vi "getCodeElementsFromApplicationXMLFile.vi"(2 "error in (no error)":errorcluster, 3 "Node":refnum<k20>) -> (0 "error out":errorcluster, 1 "TextElements":T1)   [LabVIEW 2010]
uses:
  Program Files/National Instruments/LabVIEW 2010/resource/objmgr/DOMUserDefRef.rc
panel:
  out "XML":string
  # "从应用层指令中查找出返回数据的类型、指令、控制码等信息"
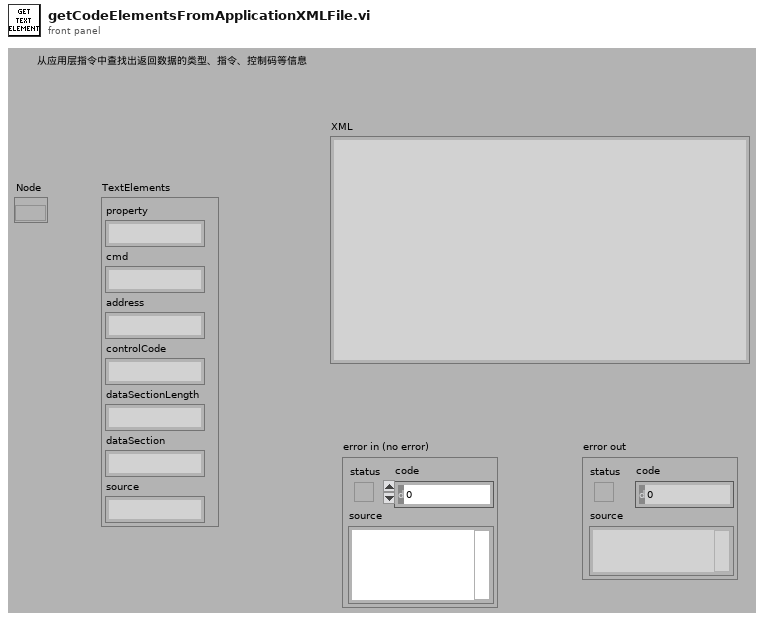
[diagram p1: front panel]
types:
  T1 = cluster{"property":string, "cmd":string, "address":string, "controlCode":string, "dataSectionLength":string, "dataSection":string, "source":string}
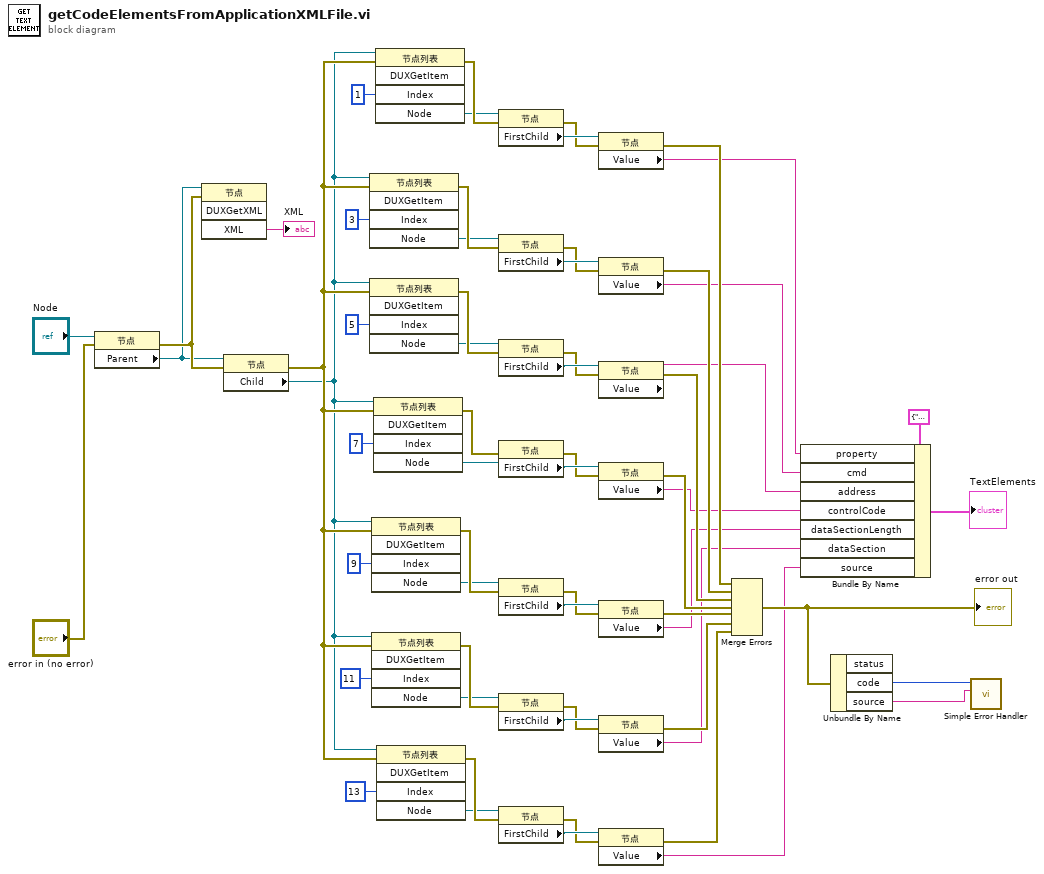
[diagram p0: block diagram]
diagram:
  n1 = property class="节点"(reference="Node", error in="error in (no error)") -> (error out=w55:errorcluster, "Parent"=w15:refnum<k20>)  [unwired: 1 out]
  n2 = invoke class="节点" method="DUXGetXML"(reference=w15, error in=w55) -> ("XML"=→"XML":string)  [unwired: 2 in, 3 out]
  n3 = property class="节点"(reference=w15, error in=w55) -> (error out=w54:errorcluster, "Child"=w22:refnum<k20>)  [unwired: 1 out]
  n4 = invoke class="节点列表" method="DUXGetItem"(reference=w22, error in=w54, "Index"=3) -> (error out=w57:errorcluster, "Node"=w24:refnum<k20>)  [unwired: 2 in, 3 out]
  n5 = invoke class="节点列表" method="DUXGetItem"(reference=w22, error in=w54, "Index"=5) -> (error out=w56:errorcluster, "Node"=w25:refnum<k20>)  [unwired: 2 in, 3 out]
  n6 = invoke class="节点列表" method="DUXGetItem"(reference=w22, error in=w54, "Index"=9) -> (error out=w59:errorcluster, "Node"=w29:refnum<k20>)  [unwired: 2 in, 3 out]
  n7 = invoke class="节点列表" method="DUXGetItem"(reference=w22, error in=w54, "Index"=11) -> (error out=w60:errorcluster, "Node"=w31:refnum<k20>)  [unwired: 2 in, 3 out]
  n8 = invoke class="节点列表" method="DUXGetItem"(reference=w22, error in=w54, "Index"=7) -> (error out=w11:errorcluster, "Node"=w27:refnum<k20>)  [unwired: 2 in, 3 out]
  n9 = invoke class="节点列表" method="DUXGetItem"(reference=w22, error in=w54, "Index"=1) -> (error out=w58:errorcluster, "Node"=w35:refnum<k20>)  [unwired: 2 in, 3 out]
  n10 = invoke class="节点列表" method="DUXGetItem"(reference=w22, error in=w54, "Index"=13) -> (error out=w61:errorcluster, "Node"=w33:refnum<k20>)  [unwired: 2 in, 3 out]
  n11 = property class="节点"(reference=w35, error in=w58) -> (error out=w10:errorcluster, "FirstChild"=w36:refnum<k20>)  [unwired: 1 out]
  n12 = property class="节点"(reference=w24, error in=w57) -> (error out=w9:errorcluster, "FirstChild"=w23:refnum<k20>)  [unwired: 1 out]
  n13 = property class="节点"(reference=w25, error in=w56) -> (error out=w8:errorcluster, "FirstChild"=w26:refnum<k20>)  [unwired: 1 out]
  n14 = property class="节点"(reference=w27, error in=w11) -> (error out=w7:errorcluster, "FirstChild"=w28:refnum<k20>)  [unwired: 1 out]
  n15 = property class="节点"(reference=w29, error in=w59) -> (error out=w6:errorcluster, "FirstChild"=w30:refnum<k20>)  [unwired: 1 out]
  n16 = property class="节点"(reference=w31, error in=w60) -> (error out=w5:errorcluster, "FirstChild"=w32:refnum<k20>)  [unwired: 1 out]
  n17 = property class="节点"(reference=w33, error in=w61) -> (error out=w4:errorcluster, "FirstChild"=w34:refnum<k20>)  [unwired: 1 out]
  n18 = property class="节点"(reference=w36, error in=w10) -> (error out=w46:errorcluster, "Value"=w38:string)  [unwired: 1 out]
  n19 = property class="节点"(reference=w23, error in=w9) -> (error out=w51:errorcluster, "Value"=w39:string)  [unwired: 1 out]
  n20 = property class="节点"(reference=w26, error in=w8) -> (error out=w50:errorcluster, "Value"=w40:string)  [unwired: 1 out]
  n21 = property class="节点"(reference=w28, error in=w7) -> (error out=w49:errorcluster, "Value"=w41:string)  [unwired: 1 out]
  n22 = property class="节点"(reference=w30, error in=w6) -> (error out=w52:errorcluster, "Value"=w42:string)  [unwired: 1 out]
  n23 = property class="节点"(reference=w32, error in=w5) -> (error out=w48:errorcluster, "Value"=w43:string)  [unwired: 1 out]
  n24 = property class="节点"(reference=w34, error in=w4) -> (error out=w47:errorcluster, "Value"=w44:string)  [unwired: 1 out]
  n25 = Merge Errors(w46, w51, w50, w49, w52, w48, w47) -> (w53:errorcluster)
  "error out" <- w53
  n26 = Bundle By Name(cluster=T1 {"property"="读通信地址", "cmd"="主站请求帧", "address"="############", "controlCode"="13", "dataSectionLength"="00", "dataSection"="无", "source"="主站"} ("TextElements"), "property"=w38, "cmd"=w39, "address"=w40, "controlCode"=w41, "dataSectionLength"=w42, "dataSection"=w43, "source"=w44) -> (→"TextElements":T1)
  n27 = Unbundle By Name(w53) -> ("code"=w1:i32, "source"=w2:string)  [unwired: 1 out]
  n28 = call <vilib>:"Simple Error Handler.vi"("error code (no error:0)"=w1, "error source (\" \")"=w2) -> ()  [unwired: 3 in, 5 out]
